vi "Set Wifi Ctrls.vi"(8 "Error In":errorcluster, 11 "NIC Info":T1) -> (0 "Error Out":errorcluster, 3 "NIC Info":T1)   [LabVIEW 2020, in "LMH-LINX.lvlib"]
uses:
  LMH-LINX.lvlib
  NIC Info.ctl
  NIC Mode.ctl
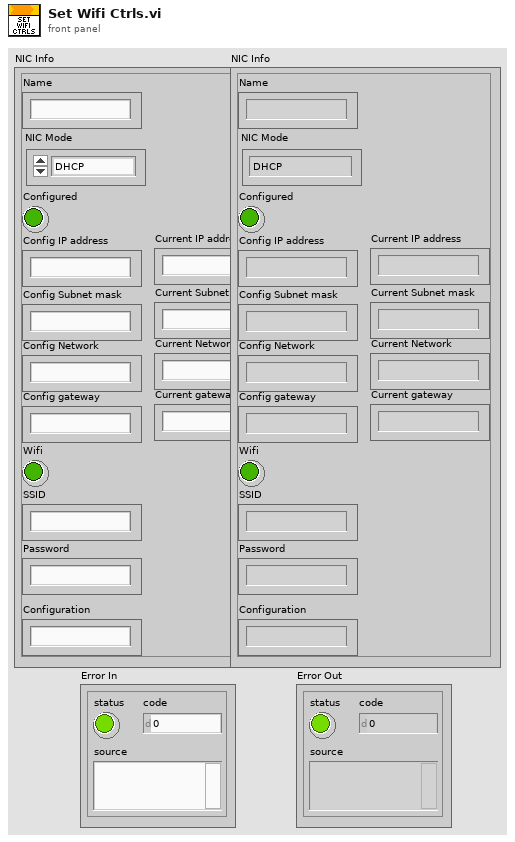
[diagram p1: front panel]
types:
  T1 = typedef "LMH-LINX.lvlib/NIC Info.ctl" = cluster{"Name":string, "NIC Mode":T2, "Configured":bool, "Config IP address":string, "Config Subnet mask":string, "Config Network":string, "Config gateway":string, "Wifi":bool, "SSID":string, "Password":string, "Configuration":string, "Current IP address":string, "Current Subnet mask":string, "Current gateway":string, "Current Network":string}
  T2 = typedef "LMH-LINX.lvlib/NIC Mode.ctl" = enum16{"DHCP", "Static", "Loopback"}
  T3 = typedef "LMH-LINX.lvlib/Network Settings Ctrl Refs.ctl" = cluster{"Hostname":refnum<vi>, "IP address":refnum<vi>, "Subnet mask":refnum<vi>, "Default Gateway":refnum<vi>, "SSID":refnum<vi>, "Password":refnum<vi>, "NIC Status":refnum<vi>, "Network Interface":refnum<vi>, "DCHP":refnum<vi>}
  T4 = enum8{"Enabled", "Disabled", "Disabled and Grayed Out"}
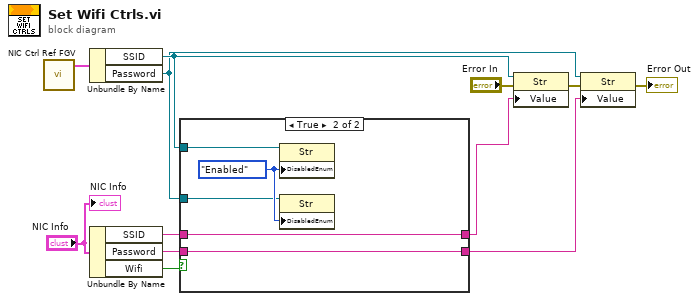
[diagram p0: block diagram]
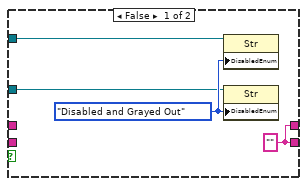
[diagram p2: hidden frame]
diagram:
  n1 = call "NIC Ctrl Ref FGV.vi"() -> ("Network Settings Ctrl Refs"=w8:T3)  [unwired: 4 in]
  n2 = Unbundle By Name(w8) -> ("SSID"=w4:refnum<vi>, "Password"=w3:refnum<vi>)
  n3 = Unbundle By Name("NIC Info") -> ("SSID"=w7:string, "Password"=w6:string, "Wifi"=w1:bool)
  n4 = case shown="True" w1 {
    tunnel: w7 -> [_ w19]
    tunnel: w6 -> [_ w21]
    tunnel: [w16 w21] -> w5
    tunnel: [w16 w19] -> w2
    tunnel: w4 -> [w14 w18]
    tunnel: w3 -> [w13 w17]
    frame False {
      w15 = T4."Disabled and Grayed Out" ("Disabled")
      w16 = "" ("SSID")
      n5 = property class="Str"(reference=w14, "DisabledEnum"=w15) -> ()  [unwired: 1 in, 2 out]
      n6 = property class="Str"(reference=w13, "DisabledEnum"=w15) -> ()  [unwired: 1 in, 2 out]
    }
    frame True {
      w20 = T4."Enabled" ("Disabled")
      n7 = property class="Str"(reference=w18, "DisabledEnum"=w20) -> ()  [unwired: 1 in, 2 out]
      n8 = property class="Str"(reference=w17, "DisabledEnum"=w20) -> ()  [unwired: 1 in, 2 out]
    }
  }
  n9 = property class="Str"(reference=w4, error in="Error In", "Value"=w2) -> (error out=w10:errorcluster)  [unwired: 1 out]
  n10 = property class="Str"(reference=w3, error in=w10, "Value"=w5) -> (error out=→"Error Out":errorcluster)  [unwired: 1 out]
  "NIC Info" <- "NIC Info"
